vi "质控参数读取.vi"(7 "section":string="氨氮质控参数", 8 "error in (no error)":errorcluster caption="错误输入（无错误）") -> (0 "error out":errorcluster caption="错误输出", 3 "参数":T1)   [LabVIEW 2016, in "质控单元.lvlib"]
uses:
  <vilib>/Utility/config.llb/Read Key (Double).vi
  <vilib>/Utility/config.llb/NI_LVConfig.lvlib
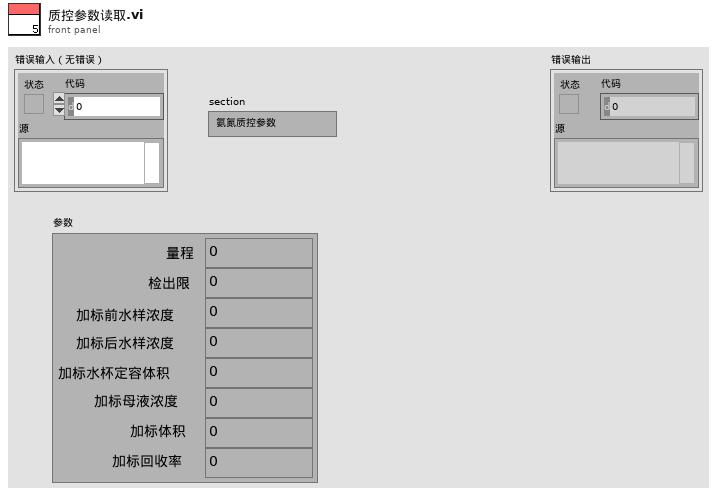
[diagram p1: front panel]
types:
  T1 = cluster{"量程":dbl, "检出限":dbl, "加标前水样浓度":dbl, "加标后水样浓度":dbl, "加标水杯定容体积":dbl, "加标母液浓度":dbl, "加标体积":dbl, "加标回收率":dbl}
  T2 = typedef "NI_LVConfig.lvlib/Config Data RefNum.ctl" = refnum<k1>
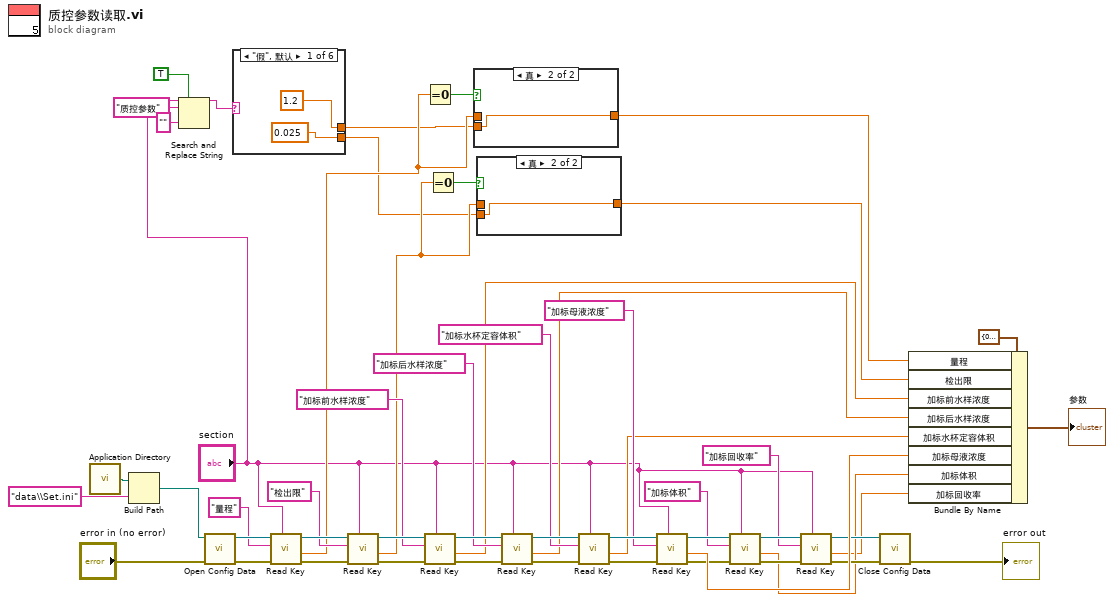
[diagram p0: block diagram]
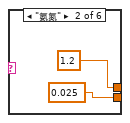
[diagram p2: hidden frame]
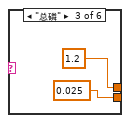
[diagram p3: hidden frame]
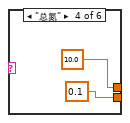
[diagram p4: hidden frame]
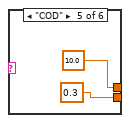
[diagram p5: hidden frame]
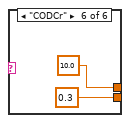
[diagram p6: hidden frame]
diagram:
  n1 = call <vilib>:"Application Directory.vi"() -> ("Application Directory"=w3:path)
  n2 = Build Path(base path=w3, name or relative path="data\\Set.ini" ("名称或相对路径")) -> (appended path=w1:path)
  n3 = Search and Replace String(replace all?=TRUE ("替换全部？(F)"), input string="section", search string="质控参数" ("搜索字符串"), replace string="" ("替换字符串(\"\")")) -> (result string=w6:string)  [unwired: 4 in, 3 out]
  n4 = call <vilib>:"Open Config Data.vi"("error in (no error)"="error in (no error)", "configuration file path"=w1) -> ("error out"=w51:errorcluster, "refnum"=w52:T2)  [unwired: 7 in, 1 out]
  n5 = case shown="\"假\", 默认" w6 {
    tunnel: [1.2 ("value") 1.2 ("value") 1.2 ("value") 10.0 ("value") 10.0 ("value") 10.0 ("value")] -> w5
    tunnel: [0.025 ("value") 0.025 ("value") 0.025 ("value") 0.1 ("value") 0.3 ("value") 0.3 ("value")] -> w4
    frame "假", Default {
    }
    frame "氨氮" {
    }
    frame "总磷" {
    }
    frame "总氮" {
    }
    frame "COD" {
    }
    frame "CODCr" {
    }
  }
  n6 = call-poly <vilib>:"Read Key.vi"("section"="section", "error in (no error)"=w51, "key"="量程", "refnum"=w52) -> ("error out"=w48:errorcluster, "value"=w15:dbl, "refnum out"=w49:T2)  [unwired: 4 in, 1 out]
  n7 = call-poly <vilib>:"Read Key.vi"("section"="section", "error in (no error)"=w48, "key"="检出限", "refnum"=w49) -> ("error out"=w46:errorcluster, "value"=w12:dbl, "refnum out"=w47:T2)  [unwired: 4 in, 1 out]
  n8 = Equal To 0?(x=w15) -> (x = 0?=w16:bool)
  n9 = call-poly <vilib>:"Read Key.vi"("section"="section", "error in (no error)"=w46, "key"="加标前水样浓度", "refnum"=w47) -> ("error out"=w40:errorcluster, "value"=w34:dbl, "refnum out"=w41:T2)  [unwired: 4 in, 1 out]
  n10 = Equal To 0?(x=w12) -> (x = 0?=w13:bool)
  n11 = case shown="真" w16 {
    tunnel: w15 -> [w65 _]
    tunnel: [w65 w66] -> w14
    tunnel: w5 -> [_ w66]
    frame False {
    }
    frame True {
    }
  }
  n12 = case shown="真" w13 {
    tunnel: w12 -> [w67 _]
    tunnel: [w67 w68] -> w11
    tunnel: w4 -> [_ w68]
    frame False {
    }
    frame True {
    }
  }
  n13 = call-poly <vilib>:"Read Key.vi"("section"="section", "error in (no error)"=w40, "key"="加标后水样浓度", "refnum"=w41) -> ("error out"=w43:errorcluster, "value"=w33:dbl, "refnum out"=w42:T2)  [unwired: 4 in, 1 out]
  n14 = call-poly <vilib>:"Read Key.vi"("section"="section", "error in (no error)"=w43, "key"="加标水杯定容体积", "refnum"=w42) -> ("error out"=w45:errorcluster, "value"=w32:dbl, "refnum out"=w44:T2)  [unwired: 4 in, 1 out]
  n15 = call-poly <vilib>:"Read Key.vi"("section"="section", "error in (no error)"=w45, "key"="加标母液浓度", "refnum"=w44) -> ("error out"=w23:errorcluster, "value"=w31:dbl, "refnum out"=w25:T2)  [unwired: 4 in, 1 out]
  n16 = call-poly <vilib>:"Read Key.vi"("section"="section", "error in (no error)"=w23, "key"="加标体积", "refnum"=w25) -> ("error out"=w22:errorcluster, "value"=w20:dbl, "refnum out"=w26:T2)  [unwired: 4 in, 1 out]
  n17 = call-poly <vilib>:"Read Key.vi"("section"="section", "error in (no error)"=w22, "key"="加标回收率", "refnum"=w26) -> ("error out"=w21:errorcluster, "value"=w19:dbl, "refnum out"=w24:T2)  [unwired: 4 in, 1 out]
  n18 = call <vilib>:"Close Config Data.vi"("error in (no error)"=w21, "refnum"=w24) -> ("error out"=→"error out":errorcluster)  [unwired: 8 in, 1 out]
  n19 = Bundle By Name(cluster=T1 {"量程"=0.0, "检出限"=0.0, "加标前水样浓度"=0.0, "加标后水样浓度"=0.0, "加标水杯定容体积"=0.0, "加标母液浓度"=0.0, "加标体积"=0.0, "加标回收率"=0.0} ("参数"), "量程"=w14, "检出限"=w11, "加标前水样浓度"=w34, "加标后水样浓度"=w33, "加标水杯定容体积"=w32, "加标母液浓度"=w31, "加标体积"=w20, "加标回收率"=w19) -> (→"参数":T1)
